vi "定位位置设置.vi"(8 "error in (no error)":errorcluster, 11 "数值":sgl) -> (0 "error out":errorcluster)   [LabVIEW 2016, in "PLC.lvlib"]
uses:
  PLC.lvlib
  <vilib>/Plasmionique/MB Master/MB_Master_Serial/MB_Master_Serial.lvclass
  C:/Program Files (x86)/National Instruments/LabVIEW 2016/vi.lib/Plasmionique/MB Master/MB_Master/MB_Master.lvclass
  <vilib>/Plasmionique/MB Master/MB Master.lvlib
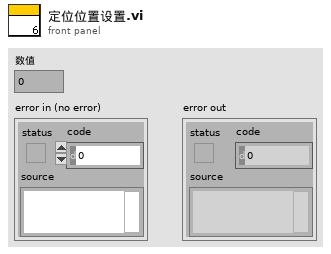
[diagram p1: front panel]
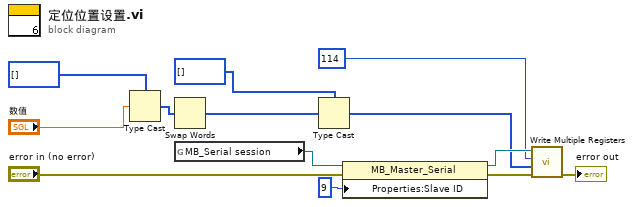
[diagram p0: block diagram]
diagram:
  n1 = Type Cast(type=u32[] [], x="数值") -> (*(type *) &x=w5:u32[])
  n2 = Swap Words(1:w5) -> (0:w4:u32[])
  n3 = global read "中间变量.vi" "MB_Serial session"() -> (w12:refnum<class "MB_Master_Serial.lvclass">)
  n4 = Type Cast(type=u16[] [], x=w4) -> (*(type *) &x=w2:u16[])
  n5 = property class="MB_Master_Serial"(reference=w12, error in="error in (no error)", "Properties:Slave ID"=u8 9 ("Slave ID")) -> (reference out=w11:refnum<class "MB_Master_Serial.lvclass">, error out=w8:errorcluster)
  n6 = call <vilib>:"Write Multiple Registers.vi"("error in (no error)"=w8, "values"=w2, "starting address"=u16 114, "MB session in"=w11) -> ("error out"=→"error out":errorcluster)  [unwired: 6 in, 1 out]
